vi "UHR-Fleezers Control (host) - 10.7.vi"() -> ()   [LabVIEW 2011] (continued)
            n774 = property on="Trap Delta (MHz)" class="DigNum (strict)"("Val(Sgnl)"="Trap Delta Before Moving") -> ()  [unwired: 2 in, 2 out]
          }
          frame #1 {
            n775 = local read "Saved Stage Positions"() -> (w1216:dbl[][])
            n776 = local write "FB Trap Pos Offset"(0.0 ("FB Trap Pos Offset")) -> ()
            n777 = property on="Trap Pos. FB Offset Factor" class="DigNum (strict)"("Val(Sgnl)"=i64 0 ("Value (Signaling)")) -> ()  [unwired: 2 in, 2 out]
            n778 = local write "Stage Moving"(TRUE ("Stage Moving")) -> ()
            n779 = call "move to saved stage position.vi"("error in"=w1213, "Stage VISA resource name in"=w1214, "Position"="Stage Position To Establish FB", "Saved Stage Positions"=w1216) -> ("error out"=w1212:errorcluster)  [unwired: 1 out]
            n780 = local write "Stage Control Serial Error"(w1212) -> ()
          }
          frame #2 {
            n781 = call <vilib>:"Beep.vi"() -> ()  [unwired: 3 in, 9 out]
            n782 = Multiply(x="Wait (s)", y=u32 1000 ("milliseconds to wait")) -> (x*y=w1222:u32)
            n783 = property on="Trap Delta (MHz)" class="DigNum (strict)"("Val(Sgnl)"="Starting \nTrap Delta (MHz)") -> ()  [unwired: 2 in, 2 out]
            n784 = local write "Stage Moving"(FALSE ("Stage Moving")) -> ()
            n785 = Wait (ms)(milliseconds to wait=w1222) -> ()  [unwired: 1 out]
            n786 = property on="Tab Control 2" class="TabCtl (strict)"("Val(Sgnl)"=T6."Feedback on Trap Position" ("Value (Signaling)")) -> ()  [unwired: 2 in, 2 out]
            n787 = property on="Tab Control" class="TabCtl (strict)"("Val(Sgnl)"=T4."Trap Control (RF)" ("Value (Signaling)")) -> ()  [unwired: 2 in, 2 out]
          }
          frame #3 {
            n788 = property on="Set Reading to\nSetpoint" class="Bool (strict)"("Val(Sgnl)"=TRUE ("Value (Signaling)")) -> ()  [unwired: 2 in, 2 out]
            n789 = Wait (ms)(milliseconds to wait=u32 500) -> ()  [unwired: 1 out]
          }
          frame #4 {
            n790 = property on="Trap Pos. FB ON" class="Bool (strict)"("Val(Sgnl)"=TRUE ("Value (Signaling)")) -> ()  [unwired: 2 in, 2 out]
            n791 = Wait (ms)(milliseconds to wait=u32 250) -> ()  [unwired: 1 out]
          }
          frame #5 {
            n792 = case shown="False" "Trap Trig Fl." {
              frame False {
                n793 = case shown="True" "Green ON after FB ON?" {
                  selector: "Green ON after FB ON?" -> [_ w1238]
                  frame False {
                  }
                  frame True {
                    n794 = property on="Green Laser ON/Interlacing" class="Bool (strict)"("Val(Sgnl)"=w1238) -> ()  [unwired: 2 in, 2 out]
                  }
                }
              }
              frame True {
              }
            }
            n795 = case shown="True" "Remove Action Offset" {
              tunnel: TRUE ("Value (Signaling)") -> [w1235 w1236]
              frame False {
                n796 = property on="Remove Unwinding Offset" class="Bool (strict)"("Val(Sgnl)"=w1235) -> ()  [unwired: 2 in, 2 out]
              }
              frame True {
                n797 = property on="Remove Action Offset" class="Bool (strict)"("Val(Sgnl)"=w1236) -> ()  [unwired: 2 in, 2 out]
              }
            }
            n798 = Wait (ms)(milliseconds to wait=u32 250) -> ()  [unwired: 1 out]
          }
          frame #6 {
            n799 = property on="Start Saving" class="Bool (strict)"("Val(Sgnl)"=TRUE ("Value (Signaling)")) -> ()  [unwired: 2 in, 2 out]
            n800 = Wait (ms)(milliseconds to wait=u32 5000) -> ()  [unwired: 1 out]
          }
          frame #7 {
            w1242 = TRUE ("Value (Signaling)")
            n801 = property on="Rem fb disp offset" class="Bool (strict)"("Val(Sgnl)"=w1242) -> ()  [unwired: 2 in, 2 out]
            n802 = property on="Remove Offset" class="Bool (strict)"("Val(Sgnl)"=w1242) -> ()  [unwired: 2 in, 2 out]
            n803 = Wait (ms)(milliseconds to wait=u32 100) -> ()  [unwired: 1 out]
          }
          frame #8 {
            n804 = case shown="True" w1245 {
              frame False {
              }
              frame True {
                n805 = local write "Trap Trig. Fl."(TRUE ("Value (Signaling)")) -> ()
              }
            }
          }
          frame #9 {
            n806 = case shown="True" "Start dipping after?" {
              frame False {
              }
              frame True {
                n807 = flat-sequence {
                  frame #0 {
                    n808 = Multiply(x="Delay before dipping (s)", y=1000.0) -> (x*y=w1249:dbl)
                    n809 = Wait (ms)(milliseconds to wait=w1249) -> ()  [unwired: 1 out]
                  }
                  frame #1 {
                    n810 = property on="Dip for Protein" class="Bool (strict)"("Val(Sgnl)"=TRUE ("Value (Signaling)")) -> ()  [unwired: 2 in, 2 out]
                    n811 = local write "Scripts"(T1."Dipping" ("Scripts")) -> ()
                  }
                }
              }
            }
          }
        }
      }
      event "Fixed Traps Data\nScript": Value Change {
        n812 = event-data() -> ()  [unwired: 1 in, 5 out]
        n813 = flat-sequence {
          frame #0 {
            n814 = case shown="True" "Green ON" {
              frame False {
              }
              frame True {
                n815 = property on="Green Laser ON/Interlacing" class="Bool (strict)"("Val(Sgnl)"=TRUE) -> ()  [unwired: 2 in, 2 out]
              }
            }
            n816 = local write "Offset (nm)"(0.0 ("Offset (nm)")) -> ()
            n817 = property on="Sample Channel\nFlow" class="Bool (strict)"("Val(Sgnl)"=FALSE ("Value (Signaling)")) -> ()  [unwired: 2 in, 2 out]
            n818 = property on="Trap Delta (MHz)" class="DigNum (strict)"("Val(Sgnl)"="Fixed Traps Trap Delta (MHz)") -> ()  [unwired: 2 in, 2 out]
          }
          frame #1 {
            n819 = Wait (ms)(milliseconds to wait=u32 1000) -> ()  [unwired: 1 out]
          }
          frame #2 {
            n820 = local write "Start Saving"(TRUE ("Start Saving")) -> ()
          }
          frame #3 {
            n821 = local read "Bead Sep. Int. Time (s)"() -> (w1260:dbl)
            n822 = Multiply(x=w1260, y=1000.0) -> (x*y=w1262:dbl)
            n823 = Wait (ms)(milliseconds to wait=w1262) -> ()  [unwired: 1 out]
          }
          frame #4 {
            n824 = property on="Remove Offset" class="Bool (strict)"("Val(Sgnl)"=TRUE ("Value (Signaling)")) -> ()  [unwired: 2 in, 2 out]
          }
          frame #5 {
            n825 = property on="Dip for Protein" class="Bool (strict)"("Val(Sgnl)"="Start dipping after?") -> ()  [unwired: 2 in, 2 out]
          }
        }
      }
      event "Got DNA bead": Value Change {
        n826 = event-data() -> ()  [unwired: 1 in, 5 out]
        n827 = flat-sequence {
          frame #0 {
            n828 = local read "Daq spot flow on"() -> (w1267:bool)
            n829 = case shown="True" w1267 {
              frame False {
              }
              frame True {
                n830 = property on="Sample Channel\nFlow" class="Bool (strict)"("Val(Sgnl)"=TRUE ("Value (Signaling)")) -> ()  [unwired: 2 in, 2 out]
              }
            }
            n831 = property on="Got DNA bead" class="Bool"("Key Focus"=FALSE) -> ()  [unwired: 2 in, 2 out]
          }
          frame #1 {
            n832 = property on="Inject Pump 1" class="Bool (strict)"("Val(Sgnl)"=FALSE ("Value (Signaling)")) -> ()  [unwired: 2 in, 2 out]
          }
          frame #2 {
            n833 = property on="Cal/Data Acq. Spot" class="Bool (strict)"("Val(Sgnl)"=TRUE ("Value (Signaling)")) -> ()  [unwired: 2 in, 2 out]
          }
        }
      }
      event "Take Stepping Data": Value Change {
        n834 = event-data() -> ()  [unwired: 1 in, 5 out]
        n835 = local read "Save ave N"() -> (w1279:dbl)
        n836 = flat-sequence {
          tunnel: w1279 -> [w1281]
          tunnel: [w1281] -> w1274
          tunnel: [w1283] -> w1275
          tunnel: w1274 -> [w1283]
          tunnel: [w1285] -> w1276
          tunnel: w1275 -> [w1285]
          tunnel: [w1288] -> w1277
          tunnel: w1276 -> [w1288]
          tunnel: [w1290] -> w1278
          tunnel: w1277 -> [w1290]
          tunnel: [w1292] -> w1272
          tunnel: w1278 -> [w1292]
          tunnel: w1272 -> [w1295]
          tunnel: [w1295] -> w1271
          tunnel: w1271 -> [w1296]
          tunnel: [w1296] -> w1273
          tunnel: w1273 -> [w1302]
          frame #0 {
            n837 = property on="Save ave N" class="DigNum (strict)"("Val(Sgnl)"="Save ave factor") -> ()  [unwired: 2 in, 2 out]
          }
          frame #1 {
            n838 = Wait (ms)(milliseconds to wait=u32 100) -> ()  [unwired: 1 out]
          }
          frame #2 {
            n839 = local read "Offset 2 Start (MHz)"() -> (w1287:dbl)
            n840 = property on="Saved AOD Raster Scan Parameter Sets" class="Arr (strict)"("Index Values"=u32[] [2]) -> ()  [unwired: 2 in, 2 out]
            n841 = property on="Trap Delta (MHz)" class="DigNum (strict)"("Val(Sgnl)"=w1287) -> ()  [unwired: 2 in, 2 out]
          }
          frame #3 {
            n842 = property on="Load parameters" class="Bool (strict)"("Val(Sgnl)"=TRUE ("Value (Signaling)")) -> ()  [unwired: 2 in, 2 out]
          }
          frame #4 {
            n843 = Wait (ms)(milliseconds to wait=u32 100) -> ()  [unwired: 1 out]
          }
          frame #5 {
            n844 = property on="Trap Raster Scan" class="Bool (strict)"("Val(Sgnl)"=TRUE ("Value (Signaling)")) -> ()  [unwired: 2 in, 2 out]
          }
          frame #6 {
            n845 = Wait (ms)(milliseconds to wait=u32 1000) -> ()  [unwired: 1 out]
          }
          frame #7 {
            n846 = while {
              stop <- w1299 stop-if-true
              n847 = local read "Raster Scanning..."() -> (w1301:bool)
              n848 = local read "Saving..."() -> (w1300:bool)
              n849 = Not(x=w1300) -> (.not. x?=w1297:bool)
              n850 = Not(x=w1301) -> (.not. x?=w1298:bool)
              n851 = And(x=w1298, y=w1297) -> (x .and. y?=w1299:bool)
            }
          }
          frame #8 {
            n852 = property on="Save ave N" class="DigNum (strict)"("Val(Sgnl)"=w1302) -> ()  [unwired: 2 in, 2 out]
          }
        }
      }
      event "Step Size (nm)": Value Change {
        n853 = event-data() -> ()  [unwired: 1 in, 5 out]
        n854 = flat-sequence {
          frame #0 {
            n855 = property on="Saved AOD Raster Scan Parameter Sets" class="Arr (strict)"("Index Values"=u32[] [1]) -> ()  [unwired: 2 in, 2 out]
          }
          frame #1 {
            n856 = Multiply(x="N Steps", y="Step Size (nm)") -> (x*y=w1304:dbl)
            n857 = property on="Scan Speed AOD (nm/s) 2" class="DigNum (strict)"("Value"="Step Size (nm)") -> ()  [unwired: 2 in, 2 out]
            n858 = property on="Step Size AOD (nm) 2" class="DigNum (strict)"("Value"="Step Size (nm)") -> ()  [unwired: 2 in, 2 out]
            n859 = property on="Scan Range AOD (nm) 2" class="DigNum (strict)"("Value"=w1304) -> ()  [unwired: 2 in, 2 out]
          }
        }
      }
      event "Take Detection Laser\nImage": Value Change {
        n860 = event-data() -> ()  [unwired: 1 in, 5 out]
        n861 = flat-sequence {
          tunnel: [w1332] -> w1322
          tunnel: [w1331] -> w1315
          tunnel: [w1330] -> w1307
          tunnel: [w1335] -> w1323
          tunnel: w1322 -> [w1335]
          tunnel: [w1334] -> w1316
          tunnel: w1315 -> [w1334]
          tunnel: [w1333] -> w1308
          tunnel: w1307 -> [w1333]
          tunnel: [w1339] -> w1324
          tunnel: w1323 -> [w1339]
          tunnel: [w1338] -> w1317
          tunnel: w1316 -> [w1338]
          tunnel: [w1337] -> w1309
          tunnel: w1308 -> [w1337]
          tunnel: [w1345] -> w1325
          tunnel: w1324 -> [w1345]
          tunnel: [w1344] -> w1318
          tunnel: w1317 -> [w1344]
          tunnel: [w1343] -> w1310
          tunnel: w1309 -> [w1343]
          tunnel: [w1349] -> w1326
          tunnel: w1325 -> [w1349]
          tunnel: [w1348] -> w1319
          tunnel: w1318 -> [w1348]
          tunnel: [w1347] -> w1311
          tunnel: w1310 -> [w1347]
          tunnel: [w1353] -> w1327
          tunnel: w1326 -> [w1353]
          tunnel: [w1352] -> w1320
          tunnel: w1319 -> [w1352]
          tunnel: [w1351] -> w1312
          tunnel: w1311 -> [w1351]
          tunnel: [w1357] -> w1328
          tunnel: w1327 -> [w1357]
          tunnel: [w1356] -> w1321
          tunnel: w1320 -> [w1356]
          tunnel: [w1355] -> w1313
          tunnel: w1312 -> [w1355]
          tunnel: w1328 -> [w1363]
          tunnel: w1321 -> [w1362]
          tunnel: [w1360] -> w1314
          tunnel: w1313 -> [w1360]
          tunnel: w1314 -> [w1364]
          frame #0 {
            n862 = local read "Green Laser ON/Interlacing"() -> (w1332:bool)
            n863 = local read "Green laser mode"() -> (w1331:enum32{"Laser ON", "Laser OFF", "Interlace"})
            n864 = local read "Green FB On/Off"() -> (w1330:bool)
          }
          frame #1 {
            n865 = property on="Green FB On/Off" class="Bool (strict)"("Val(Sgnl)"=FALSE ("Value (Signaling)")) -> ()  [unwired: 2 in, 2 out]
          }
          frame #2 {
            n866 = property on="Green Laser ON/Interlacing" class="Bool (strict)"("Val(Sgnl)"=TRUE ("Value (Signaling)")) -> ()  [unwired: 2 in, 2 out]
            n867 = property on="Flip Green Filter" class="Bool (strict)"("Val(Sgnl)"=TRUE ("Value (Signaling)")) -> ()  [unwired: 2 in, 2 out]
            n868 = property on="Green laser mode" class="RadioBtnsControl (strict)"("Val(Sgnl)"=enum32{"Laser ON", "Laser OFF", "Interlace"}."Laser ON" ("Value (Signaling)")) -> ()  [unwired: 2 in, 2 out]
          }
          frame #3 {
            n869 = Wait (ms)(milliseconds to wait=u32 500) -> ()  [unwired: 1 out]
          }
          frame #4 {
            n870 = property on="Confocal Image" class="Bool (strict)"("Val(Sgnl)"=TRUE ("Value (Signaling)")) -> ()  [unwired: 2 in, 2 out]
          }
          frame #5 {
            n871 = Wait (ms)(milliseconds to wait=u32 2000) -> ()  [unwired: 1 out]
          }
          frame #6 {
            n872 = while {
              stop <- w1358 stop-if-true
              n873 = local read "Saving..."() -> (w1359:bool)
              n874 = Not(x=w1359) -> (.not. x?=w1358:bool)
            }
          }
          frame #7 {
            n875 = property on="Flip Green Filter" class="Bool (strict)"("Val(Sgnl)"=TRUE ("Value (Signaling)")) -> ()  [unwired: 2 in, 2 out]
            n876 = property on="Green Laser ON/Interlacing" class="Bool (strict)"("Val(Sgnl)"=w1363) -> ()  [unwired: 2 in, 2 out]
            n877 = property on="Green laser mode" class="RadioBtnsControl (strict)"("Val(Sgnl)"=w1362) -> ()  [unwired: 2 in, 2 out]
          }
          frame #8 {
            n878 = property on="Green FB On/Off" class="Bool (strict)"("Val(Sgnl)"=w1364) -> ()  [unwired: 2 in, 2 out]
          }
        }
      }
      event "Stop All": Value Change {
        n879 = event-data() -> ()  [unwired: 1 in, 5 out]
        n880 = local read "Stop All"() -> (w1365:bool)
      }
    }
    n881 = node-c288() -> ()  [unwired: 1 in, 1 out]
  }
  n882 = node-c288(2 ("Processor")) -> (w92:T21)  [unwired: 3 out]
  n883 = node-c288() -> (w94:T21)  [unwired: 4 out]
  n884 = timed-loop "Control parameters (event loop)" {
    tunnel: w50 -> [w1374]
    shift-right: [w1373] -> _
    shift-left: errorcluster {"status"=FALSE, "code"=0, "source"=""} ("error out") -> [w1372]
    tunnel: [w1371] -> _
    timing: w92 -> [_]
    timing-out: [_] -> w91
    tunnel: w64 -> [w1370]
    tunnel: w4 -> [w1369]
    tunnel: w3 -> [w1368]
    tunnel: w2 -> [w1367]
    tunnel: w1 -> [w1366]
    stop <- w1371 stop-if-true
    n885 = node-c288() -> ()  [unwired: 2 out]
    n886 = event shown="[56] \"Retract Pump 3\": Value Change" {
      selector: _ -> [_ _ _ _ _ _ _ _ _ _ _ _ _ _ _ _ _ _ _ _ _ _ _ _ _ _ _ _ _ _ _ _ _ _ _ _ _ _ _ _ _ _ _ _ _ _ _ _ _ _ _ _ _ _ _ _ _ _ _ _ _ _ _ _ _ _ _ _ _ _ _ _ _]
      dyn-events: _ -> [_ _ _ _ _ _ _ _ _ _ _ _ _ _ _ _ _ _ _ _ _ _ _ _ _ _ _ _ _ _ _ _ _ _ _ _ _ _ _ _ _ _ _ _ _ _ _ _ _ _ _ _ _ _ _ _ _ _ _ _ _ _ _ _ _ _ _ _ _ _ _ _ _]
      timeout: _ -> [_ _ _ _ _ _ _ _ _ _ _ _ _ _ _ _ _ _ _ _ _ _ _ _ _ _ _ _ _ _ _ _ _ _ _ _ _ _ _ _ _ _ _ _ _ _ _ _ _ _ _ _ _ _ _ _ _ _ _ _ _ _ _ _ _ _ _ _ _ _ _ _ _]
      tunnel: w1374 -> [w1412 _ _ _ w1450 _ w1472 _ _ _ _ w1538 _ _ w1581 w1587 w1592 w1598 w1634 w1652 w1659 w1670 w1674 w1685 w1696 w1707 w1718 w1729 w1740 w1767 w1861 w1868 w1906 _ w1941 w1945 w1956 w1960 w1964 _ w1972 _ _ _ _ _ _ _ _ _ _ _ _ _ _ _ _ _ w2350 _ w2367 _ w2374 w2392 _ w2399 w2407 w2422 w2433 w2436 w2441 _ w2460]
      tunnel: [w1411 _ _ _ w1440 _ w1471 _ _ w1503 _ w1517 _ _ w1580 w1583 w1589 w1595 w1633 w1650 w1658 w1668 _ w1679 w1690 w1701 w1712 w1723 w1734 w1765 w1859 w1866 w1904 _ w1939 w1943 w1946 w1958 w1962 _ w1970 _ _ _ _ _ _ _ _ _ _ _ _ _ _ _ _ _ w2348 _ _ _ _ w2389 _ _ _ _ _ _ _ _ _] -> w1373
      tunnel: w1372 -> [w1410 _ _ _ w1449 _ w1470 _ _ w1503 _ w1537 _ _ w1579 w1582 w1588 w1594 w1632 w1651 w1657 w1669 w1673 w1684 w1695 w1706 w1717 w1728 w1739 w1766 w1860 w1867 w1905 _ w1940 w1944 w1955 w1959 w1963 _ w1971 _ _ _ _ _ _ _ _ _ _ _ _ _ _ _ _ _ w2349 _ w2366 _ w2373 w2391 _ w2398 w2406 w2421 w2432 w2435 w2440 _ w2459]
      tunnel: [_ _ _ _ _ _ _ _ _ w1502 _ _ _ _ _ _ _ _ _ _ _ _ _ _ _ _ _ _ _ _ _ _ _ _ _ _ _ _ _ _ _ _ _ _ _ _ _ _ _ _ _ _ _ _ _ _ _ _ _ _ _ _ _ _ _ _ _ _ _ _ _ _ _] -> w1371
      tunnel: [_ _ _ _ _ _ _ "Round T1 X" _ _ _ _ _ _ _ _ _ _ _ _ _ _ _ _ _ _ _ _ _ _ _ _ _ _ _ _ _ _ _ _ _ _ _ _ _ _ _ _ _ _ _ _ _ _ _ _ _ _ _ _ _ _ _ _ _ _ _ _ _ _ _ _ _] -> _
      tunnel: [_ _ _ "Adjust Scale\nto Mean" _ _ _ _ _ _ _ _ _ _ _ _ _ _ _ _ _ "Test ttrig" _ _ _ _ _ _ _ _ _ _ _ _ _ _ _ _ _ _ _ _ _ _ _ _ _ _ "Flush Sample" "Flush Pump 3" "Flush Pump 1" "Clear Volume" _ _ _ _ _ _ _ _ _ _ _ _ _ _ _ _ _ _ _ _ _] -> _
      tunnel: [_ _ _ _ _ _ _ _ "Round T2 X" _ "Delayed Interlace Start" _ _ _ _ _ _ _ _ _ _ _ _ _ _ _ _ _ _ _ _ _ _ _ _ _ _ _ _ _ _ _ _ _ _ _ _ _ _ _ _ _ _ _ _ _ _ _ _ _ _ _ _ _ _ _ _ _ _ _ _ _ _] -> _
      tunnel: w1370 -> [_ _ _ _ _ _ _ _ _ _ _ _ _ _ _ _ _ _ _ _ _ _ _ _ _ _ _ _ _ _ _ _ _ _ _ _ _ _ _ _ _ _ _ _ w2129 w2136 w2143 w2148 w2157 _ _ w2263 _ _ _ _ _ _ _ _ _ _ _ _ _ _ _ _ _ _ _ _ _]
      tunnel: w1369 -> [_ _ _ _ _ _ _ _ _ _ _ _ _ _ _ _ _ _ _ _ _ _ _ _ _ _ _ _ _ _ _ _ _ _ _ _ _ _ _ _ _ _ w2046 _ _ _ _ _ _ w2201 _ _ w2269 _ w2278 _ w2292 _ _ _ _ _ _ _ _ _ _ _ _ _ _ _ _]
      tunnel: w1368 -> [_ _ _ _ _ _ _ _ _ _ _ _ _ _ _ _ _ _ _ _ _ _ _ _ _ _ _ _ _ _ _ _ _ _ _ _ _ _ _ _ _ _ _ _ _ _ _ _ _ _ _ _ _ _ _ _ _ _ _ _ _ _ _ _ _ _ _ _ _ _ _ _ _]
      tunnel: w1367 -> [_ _ _ _ _ _ _ _ _ _ _ _ _ _ _ _ _ _ _ _ _ _ _ _ _ _ _ _ _ _ _ _ _ _ _ _ _ _ _ _ _ w1983 _ _ _ _ _ _ _ _ w2231 _ _ w2274 _ w2285 _ w2317 _ _ _ _ _ _ _ _ _ _ _ _ _ _ _]
      tunnel: w1366 -> [_ _ _ _ _ _ _ _ _ _ _ _ _ _ _ _ _ _ _ _ _ _ _ _ _ _ _ _ _ _ _ _ _ _ _ _ _ _ _ _ _ _ _ _ _ _ _ _ _ _ _ _ _ _ _ _ _ _ _ _ _ _ _ _ _ _ _ _ _ _ _ _ _]
      event "AI Count (ticks)", "Sets to FIFO (Traps)", "Save ave N", "FPGA Ave.", "# Samples/channel", "N sets to save": Value Change {
        # "So that if 'Save ave N' is updated, the AOD scanning code updates too."
        n887 = event-data() -> ()  [unwired: 6 out]
        n888 = local read "AI Count (ticks)"() -> (w1392:u32)
        n889 = Boolean To (0,1)(Boolean="Sets to FIFO (Traps)") -> (0, 1=w1402:cluster{"Set 1":i16, "Set 2":i16, "Set 3":i16})
        n890 = xnode "Read/Write Control"("FPGA VI Reference In"=w1412, "error in"=w1410, "ai count"=w1392, "AI1 Sets to FIFO"="Sets to FIFO (Traps)", "N of AI1 Int Acq Sets"="N Acq Sets (Traps + Fl.)") -> ("error out"=w1411:errorcluster)  [unwired: 1 out]
        n891 = Cluster To Array(cluster=w1402) -> (array=w1401:i16[])
        n892 = To Unsigned Long Integer(number=w1401) -> (unsigned 32bit integer=w1381:u32[])
        n893 = local read "Scan steps (AOD)"() -> (w1403:u64)
        n894 = Multiply(x=w1392, y="N Acq Sets (Traps + Fl.)") -> (x*y=w1390:u32)
        n895 = Divide(x=40000000.0, y=w1392) -> (x/y=w1384:dbl)
        "AI rate (Hz)" <- w1384
        "Ave. Rate (Hz)" <- w1384
        n896 = Add Array Elements(numeric array=w1381) -> (sum=w1393:u32)
        "Trap Sets" <- w1393
        n897 = Reciprocal(x=w1384) -> (1/x=→"Ave. Period (s)":dbl)
        n898 = property on="Scan steps (AOD)" class="DigNum (strict)"("Val(Sgnl)"=w1403) -> ()  [unwired: 2 in, 2 out]
        n899 = Divide(x=w1384, y="N Acq Sets (Traps + Fl.)") -> (x/y=w1407:dbl)
        "Data Rate (Hz)" <- w1407
        n900 = Reciprocal(x=w1407) -> (1/x=→"Data Period (s)":dbl)
        n901 = local read "Save ave N"() -> (w1406:dbl)
        n902 = Divide(x=w1407, y=w1406) -> (x/y=w1405:dbl)
        "Save Data Rate (Hz)" <- w1405
        n903 = Reciprocal(x=w1405) -> (1/x=→"Save Data Period (s)":dbl)
        n904 = Multiply(x=w1390, y="# Samples/trap") -> (x*y=w1388:u32)
        "Counts/DMA" <- w1388
        n905 = property on="Trap Disp. Downsample" class="DigNum (strict)"("Maximum"="# Samples/trap") -> ()  [unwired: 2 in, 2 out]
        n906 = Multiply(x=w1393, y="# Samples/trap") -> (x*y=w1382:u32)
        "# Samples/channel" <- w1382
        n907 = Multiply(x=w1382, y=u32 8) -> (x*y=→"Trap AI Elements/DMA read":u32)
        n908 = local read "APD Int. Count"() -> (w1389:u32)
        n909 = Multiply(x=w1382, y=u32 3) -> (x*y=→"Trap Pos Elements/DMA read":u32)
        n910 = Divide(x=w1388, y=w1389) -> (x/y=w1379:dbl)
        "APD Samples/FIFO Acq." <- w1379
        n911 = Divide(x=w1388, y=40000000.0) -> (x/y=w1386:dbl)
        "DMA Update Period (s)" <- w1386
        n912 = Multiply(x=2.0, y=w1379) -> (x*y=→"APD Elements/DMA read":dbl)
        n913 = property on="APD Disp. Downsample" class="DigNum (strict)"("Maximum"=w1379) -> ()  [unwired: 2 in, 2 out]
        n914 = local read "N sets to save"() -> (w1399:u32)
        n915 = Multiply(x=w1386, y=w1399) -> (x*y=→"Total Time (s)":dbl)
        "FPGA Averaging" <- FALSE ("FPGA Averaging")
      }
      event "Remove Offset": Value Change {
        n916 = event-data() -> ()  [unwired: 7 out]
        n917 = local write "Remove Offset"(FALSE ("Remove Offset")) -> ()
        n918 = local read "Bead Mean (nm)"() -> (w1414:dbl)
        n919 = local read "Offset (nm)"() -> (w1415:dbl)
        n920 = Add(x=w1414, y=w1415) -> (x+y=w1413:dbl)
        n921 = local write "Offset (nm)"(w1413) -> ()
        n922 = disable-structure shown="Disabled" {
          frame Disabled {
            n923 = local read "Bead Mean (nm)"() -> (w1420:dbl)
            n924 = Add(y=w1420) -> (x=w1419:dbl, x+y=w1418:dbl)
            n925 = Subtract(x=w1420, y=w1419) -> (x-y=w1417:dbl)
            n926 = property on="Bead Separation" class="WFChart (strict)"("YScale.Minimum"=w1417) -> ()  [unwired: 2 in, 2 out]
            n927 = property on="Bead Separation" class="WFChart (strict)"("YScale.Maximum"=w1418) -> ()  [unwired: 2 in, 2 out]
          }
          frame Enabled {
          }
        }
      }
      event "Detector Type": Value Change {
        n928 = event-data() -> ()  [unwired: 7 out]
        n929 = local read "AI labels"() -> (w1421:string[])
        n930 = property on="High Res. Display" class="Ring (strict)"("Strings []"=w1421) -> ()  [unwired: 2 in, 2 out]
        n931 = Build Array (concatenate)(w1421, "none") -> (w1422:string[])
        n932 = property on="FFT 1 Choice 1" class="Ring (strict)"("Strings []"=w1422) -> ()  [unwired: 2 in, 2 out]
        n933 = property on="FFT 1 Choice 2" class="Ring (strict)"("Strings []"=w1422) -> ()  [unwired: 2 in, 2 out]
        n934 = property on="FFT 2 Choice 1" class="Ring (strict)"("Strings []"=w1422) -> ()  [unwired: 2 in, 2 out]
        n935 = property on="FFT 2 Choice 2" class="Ring (strict)"("Strings []"=w1422) -> ()  [unwired: 2 in, 2 out]
        n936 = Bundle("APD 1", "APD 2") -> (w1425:cluster{string, string})  [unwired: 1 out]
        n937 = Cluster To Array(cluster=w1425) -> (array=w1423:string[])
        n938 = Build Array (concatenate)(w1423, w1422) -> (w1427:string[])
        n939 = Array Size(array=w1427) -> (size(s)=w1428:i32)
        n940 = property on="Signals to Plot" class="LstBox (strict)"("Item Names"=w1427) -> ()  [unwired: 2 in, 2 out]
        n941 = property on="Signals to Plot" class="LstBox (strict)"("Number of Rows"=w1428) -> ()  [unwired: 2 in, 2 out]
        n942 = property on="All Signals" class="WFChart (strict)"("LegNumRows"=w1428) -> ()  [unwired: 2 in, 2 out]
      }
      event "Adjust Scale\nto Mean": Value Change {
        n943 = event-data() -> ()  [unwired: 7 out]
        n944 = local read "APD 1 Rate (Hz)"() -> (w1437:dbl)
        n945 = Multiply(x=1000.0, y="Above (kHz)") -> (x*y=w1435:dbl)
        n946 = Multiply(x=1000.0, y="Below (kHz)") -> (x*y=w1433:dbl)
        n947 = Add(x=w1435, y=w1437) -> (x+y=w1430:dbl)
        n948 = Subtract(x=w1437, y=w1433) -> (x-y=w1431:dbl)
        n949 = property on="APD Chart" class="WFChart (strict)"("YScale.Minimum"=w1431) -> ()  [unwired: 2 in, 2 out]
        n950 = property on="APD Chart" class="WFChart (strict)"("YScale.Maximum"=w1430) -> ()  [unwired: 2 in, 2 out]
      }
      event "Phase adj. (AI1)", "+ phase (AI1)", "- phase (AI1)": Value Change {
        n951 = event-data() -> ()  [unwired: 7 out]
        n952 = Negate(x="Phase adj. (AI1)") -> (-x=w1447:i16)
        n953 = Select(t=w1447, s="- phase (AI1)", f="Phase adj. (AI1)") -> (s? t:f=w1446:i16)
        n954 = xnode "Read/Write Control"("FPGA VI Reference In"=w1450, "error in"=w1449, "Phase count adjustment"=w1446) -> ("FPGA VI Reference Out"=w1445:T19, "error out"=w1444:errorcluster)
        n955 = Or(x="- phase (AI1)", y="+ phase (AI1)") -> (x .or. y?=w1441:bool)
        n956 = xnode "Read/Write Control"("FPGA VI Reference In"=w1445, "error in"=w1444, "+ phase"=w1441) -> ("error out"=w1440:errorcluster)  [unwired: 1 out]
      }
      event "Signals to Plot": Double Click {
        w1453 = u32 9868950 ("Color Box")
        n957 = event-data() -> ("Row"=w1455:i32)  [unwired: 9 out]
        n958 = property on="All Signals" class="WFChart (strict)"("Active Plot"=w1455) -> (error out=w1466:errorcluster)  [unwired: 2 in, 1 out]
        n959 = property on="All Signals" class="WFChart (strict)" props=["Plot", "Visible?", "Plot", "Plot Color"](error in=w1466) -> (error out=w1465:errorcluster, "Plot.Visible?"=w1464:bool)  [unwired: 1 in, 2 out]
        n960 = Select(t=FALSE ("Plot.Visible"), s=w1464, f=TRUE ("Plot.Visible")) -> (s? t:f=w1459:bool)
        n961 = property on="All Signals" class="WFChart (strict)"(error in=w1465, "Plot.Visible?"=w1459) -> (error out=w1461:errorcluster)  [unwired: 1 in, 1 out]
        n962 = property on="All Signals" class="WFChart (strict)"(error in=w1461) -> (error out=w1456:errorcluster, "Plot.Plot Color"=w1460:u32)  [unwired: 1 in, 1 out]
        n963 = property on="Signals to Plot" class="LstBox (strict)"(error in=w1456, "Active Row"=w1455) -> (error out=w1454:errorcluster)  [unwired: 1 in, 1 out]
        n964 = Select(t=w1460, s=w1459, f=u32 0) -> (s? t:f=w1457:u32)
        n965 = property on="Signals to Plot" class="LstBox (strict)"(error in=w1454, "CellFontColor"=w1457, "SelColor"=w1453, "CellBG"=w1453, "CellFontSize"=u32 20 ("Active Row:Cell Font:Size"), "CellFontBold"=TRUE ("Active Row:Cell Font:Bold")) -> ()  [unwired: 1 in, 2 out]
      }
      event "BD 1 Frequency 1 (MHz)", "BD 1 Frequency 2 (MHz)", "BD 1 Frequency 3 (MHz)", "BD 2 Frequency 1 (MHz)", "BD 2 Frequency 2 (MHz)", "BD 2 Frequency 3 (MHz)", "Trap Delta (MHz)": Value Change {
        n966 = event-data() -> ("CtlRef"=w1469:refnum<vi>)  [unwired: 6 out]
        n967 = control-ref of="Trap Delta (MHz)"() -> (w1468:refnum<vi>)
        n968 = Equal?(x=w1468, y=w1469) -> (x = y?=w1467:bool)
        n969 = case shown="False" "Oscillate Set 1" {
          tunnel: w1472 -> [w1492 _]
          tunnel: [w1491 w1495] -> w1471
          tunnel: w1470 -> [w1490 w1495]
          tunnel: w1467 -> [w1475 _]
          frame False {
            n970 = local read "BD 1 Frequency 2 (MHz)"() -> (w1479:dbl)
            n971 = local read "BD 1 Frequency 1 (MHz)"() -> (w1477:dbl)
            n972 = Subtract(x=w1479, y="Trap Delta (MHz)") -> (x-y=w1476:dbl)
            n973 = Select(t=w1476, s=w1475, f=w1477) -> (s? t:f=w1474:dbl)
            n974 = local read "Y RF Frequency Limits (MHz)"() -> (w1480:T16)
            n975 = local read "X RF Frequency Limits (MHz)"() -> (w1481:T16)
            n976 = local read "BD 1 Frequency 3 (MHz)"() -> (w1493:dbl)
            n977 = local write "BD 1 Frequency 1 (MHz)"(w1474) -> ()
            n978 = local read "BD 2 Frequency 1 (MHz)"() -> (w1484:dbl)
            n979 = local read "BD 2 Frequency 2 (MHz)"() -> (w1483:dbl)
            n980 = local read "BD 2 Frequency 3 (MHz)"() -> (w1494:dbl)
            n981 = call "set RF board frequency - interlace.vi"("Board 2 Frequency Limits"=w1480, "Board 1 Frequency Limits"=w1481, "error in"=w1490, "FPGA VI Reference In"=w1492, "Board 2 Frequency 3 (MHz)"=w1494, "Board 1 Frequency 3 (MHz)"=w1493, "Board 2 Frequency 2 (MHz)"=w1483, "Board 2 Frequency 1 (MHz)"=w1484, "Board 1 Frequency 2 (MHz)"=w1479, "Board 1 Frequency 1  (MHz)"=w1474) -> ("error out"=w1491:errorcluster)  [unwired: 1 out]
            n982 = Subtract(x=w1484, y=w1483) -> (x-y=w1488:dbl)
            n983 = Subtract(x=w1474, y=w1479) -> (x-y=w1489:dbl)
            n984 = Square(x=w1488) -> (x^2=w1486:dbl)
            n985 = Square(x=w1489) -> (x^2=w1487:dbl)
            n986 = Add(x=w1487, y=w1486) -> (x+y=w1485:dbl)
            n987 = Square Root(x=w1485) -> (sqrt(x)=w1482:dbl)
            n988 = local write "Trap Delta (MHz)"(w1482) -> ()
            n989 = property on="Initial delta (MHz)" class="DigNum (strict)"("Val(Sgnl)"=w1482) -> ()  [unwired: 2 in, 2 out]
          }
          frame True {
          }
        }
      }
      event "Round T1 X": Value Change {
        n990 = event-data() -> ()  [unwired: 7 out]
        n991 = local read "BD 1 Frequency 1 (MHz)"() -> (w1498:dbl)
        n992 = Round To Nearest(number=w1498) -> (nearest integer value=w1497:dbl)
        n993 = property on="BD 1 Frequency 1 (MHz)" class="DigNum (strict)"("Val(Sgnl)"=w1497) -> ()  [unwired: 2 in, 2 out]
      }
      event "Round T2 X": Value Change {
        n994 = event-data() -> ()  [unwired: 7 out]
        n995 = local read "BD 1 Frequency 2 (MHz)"() -> (w1500:dbl)
        n996 = Round To Nearest(number=w1500) -> (nearest integer value=w1499:dbl)
        n997 = property on="BD 1 Frequency 2 (MHz)" class="DigNum (strict)"("Val(Sgnl)"=w1499) -> ()  [unwired: 2 in, 2 out]
      }
      event "Stop All": Value Change {
        n998 = event-data() -> ()  [unwired: 7 out]
        n999 = local read "Stop All"() -> (w1502:bool)
      }
      event "Delayed Interlace Start": Value Change {
        n1000 = event-data() -> ()  [unwired: 7 out]
        n1001 = flat-sequence {
          frame #0 {
            n1002 = Multiply(x="Delay to Interlace (s)", y=1000.0) -> (x*y=w1505:dbl)
            n1003 = Wait (ms)(milliseconds to wait=w1505) -> ()  [unwired: 1 out]
          }
          frame #1 {
            n1004 = property on="Green laser mode" class="RadioBtnsControl (strict)"("Val(Sgnl)"=enum32{"Laser ON", "Laser OFF", "Interlace"}."Interlace" ("Value (Signaling)")) -> ()  [unwired: 2 in, 2 out]
          }
        }
      }
      event "BD 1 Amplitude 1 (%)", "BD 1 Amplitude 2 (%)", "BD 1 Amplitude 3 (%)", "BD 2 Amplitude 1 (%)", "BD 2 Amplitude 2 (%)", "BD 2 Amplitude 3 (%)", "Trap 1 ON", "Trap 2 ON", "Trap 3 ON", "Feedback On/Off", "All FB On/Off": Value Change {
        w1529 = i16 1 ("f")
        n1005 = event-data() -> ()  [unwired: 7 out]
        n1006 = local write "Trap 1 (ON/OFF)"("Trap 1 ON") -> ()
        n1007 = local write "Trap 2 (ON/OFF)"("Trap 2 ON") -> ()
        n1008 = Boolean To (0,1)(Boolean="Trap 3 ON") -> (0, 1=w1530:i16)
        n1009 = Boolean To (0,1)(Boolean="Trap 1 ON") -> (0, 1=w1531:i16)
        n1010 = Boolean To (0,1)(Boolean="Trap 2 ON") -> (0, 1=w1532:i16)
        n1011 = Select(t=w1532, s="Trap ON/OFF X or Y Amp?", f=w1529) -> (s? t:f=w1527:i16)
        n1012 = Select(t=w1531, s="Trap ON/OFF X or Y Amp?", f=w1529) -> (s? t:f=w1528:i16)
        n1013 = Select(t=w1530, s="Trap ON/OFF X or Y Amp?", f=w1529) -> (s? t:f=w1526:i16)
        n1014 = Select(t=w1529, s="Trap ON/OFF X or Y Amp?", f=w1532) -> (s? t:f=w1524:i16)
        n1015 = Select(t=w1529, s="Trap ON/OFF X or Y Amp?", f=w1531) -> (s? t:f=w1525:i16)
        n1016 = Select(t=w1529, s="Trap ON/OFF X or Y Amp?", f=w1530) -> (s? t:f=w1523:i16)
        n1017 = And(x="All FB On/Off", y="Feedback On/Off") -> (x .and. y?=w1521:cluster{"Set 1":bool, "Set 2":bool})
        n1018 = local read "BD 1 Amplitude 1 (%)"() -> (w1541:dbl)
        n1019 = local read "BD 1 Amplitude 2 (%)"() -> (w1540:dbl)
        n1020 = local read "BD 1 Amplitude 3 (%)"() -> (w1539:dbl)
        n1021 = Unbundle By Name(w1521) -> ("Set 1"=w1516:bool, "Set 2"=w1513:bool)
        n1022 = local read "Y RF Amplitude Limits (%)"() -> (w1509:T16)
        n1023 = local read "X RF Amplitude Limits (%)"() -> (w1510:T16)
        n1024 = local read "BD 2 Amplitude 1 (%)"() -> (w1542:dbl)
        n1025 = local read "BD 2 Amplitude 2 (%)"() -> (w1543:dbl)
        n1026 = local read "BD 2 Amplitude 3 (%)"() -> (w1544:dbl)
        n1027 = And(x="Trap 2 ON", y=w1513) -> (x .and. y?=w1511:bool)
        n1028 = And(x="Trap 1 ON", y=w1516) -> (x .and. y?=w1514:bool)
        n1029 = Multiply(x=w1528, y=w1541) -> (x*y=w1536:dbl)
        n1030 = Multiply(x=w1540, y=w1527) -> (x*y=w1534:dbl)
        n1031 = Multiply(x=w1539, y=w1526) -> (x*y=w1535:dbl)
        n1032 = Multiply(x=w1542, y=w1525) -> (x*y=w1545:dbl)
        n1033 = Multiply(x=w1543, y=w1524) -> (x*y=w1546:dbl)
        n1034 = Multiply(x=w1544, y=w1523) -> (x*y=w1547:dbl)
        n1035 = call "set RF board amplitude - interlace.vi"("Board 2 Amplitude Limits"=w1509, "Board 1 Amplitude Limits"=w1510, "error in"=w1537, "FPGA VI Reference In"=w1538, "Board 2 Amplitude 3 (%)"=w1547, "Board 1 Amplitude 3 (%)"=w1535, "Board 2 Amplitude 2 (%)"=w1546, "Board 2 Amplitude 1 (%)"=w1545, "Board 1 Amplitude 2 (%)"=w1534, "Board 1 Amplitude 1 (%)"=w1536) -> ("error out"=w1518:errorcluster, "FPGA VI Reference Out"=w1519:T19)
        n1036 = xnode "Read/Write Control"("FPGA VI Reference In"=w1519, "error in"=w1518, "FB On/Off Set 1"=w1514, "FB On/Off Set 2"=w1511) -> ("error out"=w1517:errorcluster)  [unwired: 1 out]
      }
      event "Load parameters": Value Change {
        n1037 = event-data() -> ()  [unwired: 7 out]
        n1038 = property on="Saved AOD Raster Scan Parameter Sets" class="Arr (strict)"() -> ("Index Values"=w1558:u32[])  [unwired: 2 in, 2 out]
        n1039 = Index Array(array=w1558, index=0) -> (element=w1555:u32)
        n1040 = local write "Load parameters"(FALSE ("Load parameters")) -> ()
        n1041 = Index Array(array="Saved AOD Raster Scan Parameter Sets", index=w1555) -> (element=w1554:T26)
        n1042 = Unbundle By Name(w1554) -> ("Scan Range AOD (nm) 2"=w1553:dbl, "Step Size AOD (nm) 2"=w1552:dbl, "Scan Speed AOD (nm/s) 2"=w1551:dbl, "Number of scans (AOD) 2"=w1550:u16)
        n1043 = flat-sequence {
          tunnel: w1553 -> [w1561]
          tunnel: w1552 -> [w1560]
          tunnel: w1551 -> [w1559]
          tunnel: w1550 -> [w1562]
          frame #0 {
            n1044 = local write "Scan Speed (nm/s)"(w1559) -> ()
            n1045 = local write "Scan Range (nm)"(w1561) -> ()
            n1046 = local write "Step Size (nm)"(w1560) -> ()
          }
          frame #1 {
            n1047 = property on="Number of F/B Scans (AOD)" class="DigNum (strict)"("Val(Sgnl)"=w1562) -> ()  [unwired: 2 in, 2 out]
          }
        }
      }
      event "Trap 1 (ON/OFF)", "Trap 2 (ON/OFF)": Value Change {
        n1048 = event-data() -> ()  [unwired: 7 out]
        n1049 = property on="Trap 2 ON" class="Bool (strict)"("Val(Sgnl)"="Trap 2 (ON/OFF)") -> ()  [unwired: 2 in, 2 out]
        n1050 = property on="Trap 1 ON" class="Bool (strict)"("Val(Sgnl)"="Trap 1 (ON/OFF)") -> ()  [unwired: 2 in, 2 out]
      }
      event "DIO count 1 (ticks)", "DIO count 2 (ticks)", "DIO count 3 (ticks)", "Interlace", "Number Interlace Sets", "Not-Interlacing Set": Value Change {
        n1051 = event-data() -> ()  [unwired: 7 out]
        n1052 = local read "DIO count 3 (ticks)"() -> (w1575:u32)
        n1053 = local read "DIO count 1 (ticks)"() -> (w1577:u32)
        n1054 = local read "DIO count 2 (ticks)"() -> (w1576:u32)
        n1055 = To Unsigned Byte Integer(number="Not-Interlacing Set") -> (unsigned 8bit integer=w1566:u8)
        n1056 = Add(x=w1566, y=u8 1) -> (x+y=w1570:u8)
        n1057 = xnode "Read/Write Control"("FPGA VI Reference In"=w1581, "error in"=w1579, "DIO count 1 (ticks)"=w1577, "DIO count 2 (ticks)"=w1576, "DIO count 3 (ticks)"=w1575, "Interlace ON/OFF"="Interlace", "Number Interlace Cycles"="Number Interlace Sets", "Interlace Off Parameters"=w1570) -> ("error out"=w1580:errorcluster)  [unwired: 1 out]
        n1058 = Build Array(w1577, w1576, w1575) -> (w1568:u32[])
        n1059 = Split 1D Array(array=w1568, index="Number Interlace Sets") -> (first subarray=w1578:u32[])  [unwired: 1 out]
        n1060 = Index Array(array=w1568, index=w1566) -> (element=w1567:u32)
        n1061 = Add Array Elements(numeric array=w1578) -> (sum=w1572:u32)
        n1062 = Select(t=w1572, s="Interlace", f=w1567) -> (s? t:f=→"Total Counts (ticks)":u32)
      }
      event "Reset Feedback": Value Change {
        n1063 = event-data() -> ()  [unwired: 7 out]
        n1064 = Unbundle By Name("Reset Feedback") -> ("Set 1"=w1585:bool, "Set 2"=w1584:bool)
        n1065 = xnode "Read/Write Control"("FPGA VI Reference In"=w1587, "error in"=w1582, "FB Reset Set 1"=w1585, "FB Reset Set 2"=w1584) -> ("error out"=w1583:errorcluster)  [unwired: 1 out]
      }
      event "PID Gains": Value Change {
        n1066 = event-data() -> ()  [unwired: 7 out]
        n1067 = Unbundle By Name("PID Gains") -> ("Set 1"=w1591:T14, "Set 2"=w1590:T14)
        n1068 = xnode "Read/Write Control"("FPGA VI Reference In"=w1592, "error in"=w1588, "FB Gains Set 1"=w1591, "FB Gains Set 2"=w1590) -> ("error out"=w1589:errorcluster)  [unwired: 1 out]
      }
      event "AI2 to Setpoint", "Setpoints (V)": Value Change {
        n1069 = event-data() -> ()  [unwired: 7 out]
        n1070 = xnode "Read/Write Control"("FPGA VI Reference In"=w1598, "error in"=w1594) -> ("FPGA VI Reference Out"=w1597:T19, "error out"=w1596:errorcluster, "AI2 Y Sum Set 1"=w1605:i16, "AI2 Y Sum Set 2"=w1604:i16)
        n1071 = Cluster To Array(cluster="AI2 to Setpoint") -> (array=w1608:bool[])
        n1072 = local read "AI2 (V)"() -> (w1606:cluster{"Set 1":dbl, "Set 2":dbl})
        n1073 = Or Array Elements(Boolean array=w1608) -> (logical OR=w1609:bool)
        n1074 = Bundle By Name(cluster=w1606, "Set 1"=w1605, "Set 2"=w1604) -> (w1603:cluster{"Set 1":dbl, "Set 2":dbl})
        n1075 = Divide(x=w1603, y=3276.7) -> (x/y=w1602:cluster{"Set 1":dbl, "Set 2":dbl})
        "AI2 (V)" <- w1602
        n1076 = case shown="True" w1609 {
          tunnel: [w1612 w1629] -> w1601
          tunnel: "AI2 to Setpoint" -> [_ w1625]
          tunnel: "Setpoints (V)" -> [w1613 w1628]
          tunnel: w1602 -> [_ w1622]
          frame False {
            n1077 = Multiply(x=3276.7, y=w1613) -> (x*y=w1614:cluster{"Set 1":dbl, "Set 2":dbl})
            n1078 = To Word Integer(number=w1614) -> (16bit integer=w1612:cluster{"Set 1":i16, "Set 2":i16})
          }
          frame True {
            n1079 = Unbundle By Name(w1622) -> ("Set 1"=w1621:dbl, "Set 2"=w1620:dbl)
            n1080 = Unbundle By Name(w1628) -> ("Set 1"=w1627:dbl, "Set 2"=w1626:dbl)
            n1081 = Unbundle By Name(w1625) -> ("Set 1"=w1624:bool, "Set 2"=w1623:bool)
            n1082 = Select(t=w1621, s=w1624, f=w1627) -> (s? t:f=w1619:dbl)
            n1083 = Select(t=w1620, s=w1623, f=w1626) -> (s? t:f=w1618:dbl)
            n1084 = Bundle By Name(cluster=w1628, "Set 1"=w1619, "Set 2"=w1618) -> (w1616:cluster{"Set 1":dbl, "Set 2":dbl})
            n1085 = local write "Setpoints (V)"(w1616) -> ()
            n1086 = Multiply(x=3276.7, y=w1616) -> (x*y=w1617:cluster{"Set 1":dbl, "Set 2":dbl})
            n1087 = To Word Integer(number=w1617) -> (16bit integer=w1629:cluster{"Set 1":i16, "Set 2":i16})
          }
        }
        n1088 = Unbundle By Name(w1601) -> ("Set 1"=w1600:i16, "Set 2"=w1599:i16)
        n1089 = xnode "Read/Write Control"("FPGA VI Reference In"=w1597, "error in"=w1596, "FB Setpoint Set 1"=w1600, "FB Setpoint Set 2"=w1599) -> ("error out"=w1595:errorcluster)  [unwired: 1 out]
      }
      event "Invert GI": Value Change {
        n1090 = event-data() -> ()  [unwired: 7 out]
        n1091 = xnode "Read/Write Control"("FPGA VI Reference In"=w1634, "error in"=w1632, "Invert GI"="Invert GI", "Invert GI 2"="Invert GI") -> ("error out"=w1633:errorcluster)  [unwired: 1 out]
      }
      event "Green FB Setpoint (mV)", "Green FB Gains", "Green FB On/Off", "Current When FB OFF (%)", "Green int current ON count adj": Value Change {
        n1092 = event-data() -> ()  [unwired: 7 out]
        n1093 = local read "Green FB Setpoint (mV)"() -> (w1641:dbl)
        n1094 = local read "Current When FB OFF (%)"() -> (w1644:dbl)
        n1095 = Multiply(x=w1641, y=3.2767) -> (x*y=w1640:dbl)
        n1096 = Multiply(x=w1644, y=655.35) -> (x*y=w1645:dbl)
        n1097 = To Unsigned Word Integer(number=w1645) -> (unsigned 16bit integer=w1643:u16)
        n1098 = local read "Green int current ON count adj"() -> (w1648:u32)
        n1099 = local read "Green FB Gains"() -> (w1647:T14)
        n1100 = local read "Green Laser ON/Interlacing"() -> (w1638:bool)
        n1101 = local read "Green laser mode"() -> (w1637:enum32{"Laser ON", "Laser OFF", "Interlace"})
        n1102 = local read "Green FB On/Off"() -> (w1649:bool)
        n1103 = Equal?(x=w1637, y=enum32{"Laser ON", "Laser OFF", "Interlace"}."Interlace") -> (x = y?=w1635:bool)
        n1104 = Compound Arithmetic op=AND(w1635, w1649, w1638) -> (w1639:bool)
        n1105 = xnode "Read/Write Control"("FPGA VI Reference In"=w1652, "error in"=w1651, "Green FB Setpoint"=w1640, "Green FB On/Off"=w1639, "Current Out"=w1643, "Green int current ON count adj"=w1648, "Green FB Gains"=w1647) -> ("error out"=w1650:errorcluster)  [unwired: 1 out]
      }
      event "Green laser mode", "Green Laser ON/Interlacing": Value Change {
        n1106 = event-data() -> ()  [unwired: 7 out]
        n1107 = case shown="True" "Green Laser ON/Interlacing" {
          tunnel: "Green laser mode" -> [_ w1666]
          tunnel: [enum32{"Laser ON", "Laser OFF", "Interlace"}."Laser OFF" ("Green laser mode") w1666] -> w1654
          tunnel: [FALSE w1662] -> w1653
          frame False {
          }
          frame True {
            n1108 = local read "Green FB On/Off"() -> (w1663:bool)
            n1109 = Equal?(x=w1666, y=enum32{"Laser ON", "Laser OFF", "Interlace"}."Interlace") -> (x = y?=w1664:bool)
            n1110 = And(x=w1664, y=w1663) -> (x .and. y?=w1662:bool)
          }
        }
        n1111 = xnode "Read/Write Control"("FPGA VI Reference In"=w1659, "error in"=w1657, "Operating Mode"=w1654, "Operating Mode 2"=w1654, "Green FB On/Off"=w1653) -> ("error out"=w1658:errorcluster)  [unwired: 1 out]
      }
      event "Test ttrig": Value Change {
        n1112 = event-data() -> ()  [unwired: 7 out]
        n1113 = xnode "Read/Write Control"("FPGA VI Reference In"=w1670, "error in"=w1669, "TTrig?"=TRUE) -> ("error out"=w1668:errorcluster)  [unwired: 1 out]
      }
      event "Neg. TTrig FPGA": Value Change {
        n1114 = event-data() -> ()  [unwired: 7 out]
        n1115 = xnode "Read/Write Control"("FPGA VI Reference In"=w1674, "error in"=w1673, "TTrig Negate Pos"="Neg. TTrig FPGA") -> ()  [unwired: 2 out]
      }
      event "- phase (APD 1 Gate)", "+ phase (APD 1 Gate)": Value Change {
        n1116 = event-data() -> ()  [unwired: 7 out]
        n1117 = local read "Phase Adj. (APD 1 Gate)"() -> (w1675:i16)
        n1118 = Negate(x=w1675) -> (-x=w1683:i16)
        n1119 = Select(t=w1683, s="- phase (APD 1 Gate)", f=w1675) -> (s? t:f=w1682:i16)
        n1120 = Or(x="- phase (APD 1 Gate)", y="+ phase (APD 1 Gate)") -> (x .or. y?=w1678:bool)
        n1121 = xnode "Read/Write Control"("FPGA VI Reference In"=w1685, "error in"=w1684, "Phase count adjustment (APD 1 Gate)"=w1682) -> ("FPGA VI Reference Out"=w1680:T19, "error out"=w1681:errorcluster)
        n1122 = xnode "Read/Write Control"("FPGA VI Reference In"=w1680, "error in"=w1681, "+ phase (APD 1 Gate)"=w1678) -> ("error out"=w1679:errorcluster)  [unwired: 1 out]
      }
      event "+ phase (APD 2 Gate)", "- phase (APD 2 Gate)": Value Change {
        n1123 = event-data() -> ()  [unwired: 7 out]
        n1124 = local read "Phase Adj. (APD 2 Gate)"() -> (w1686:i16)
        n1125 = Negate(x=w1686) -> (-x=w1694:i16)
        n1126 = Select(t=w1694, s="- phase (APD 2 Gate)", f=w1686) -> (s? t:f=w1693:i16)
        n1127 = Or(x="- phase (APD 2 Gate)", y="+ phase (APD 2 Gate)") -> (x .or. y?=w1689:bool)
        n1128 = xnode "Read/Write Control"("FPGA VI Reference In"=w1696, "error in"=w1695, "Phase count adjustment (APD 2 Gate)"=w1693) -> ("FPGA VI Reference Out"=w1691:T19, "error out"=w1692:errorcluster)
        n1129 = xnode "Read/Write Control"("FPGA VI Reference In"=w1691, "error in"=w1692, "+ phase (APD 2 Gate)"=w1689) -> ("error out"=w1690:errorcluster)  [unwired: 1 out]
      }
      event "Phase Adj. (APD Acq)", "+ phase (APD Acq)", "- phase (APD Acq)": Value Change {
        n1130 = event-data() -> ()  [unwired: 7 out]
        n1131 = local read "Phase Adj. (APD Acq)"() -> (w1699:i16)
        n1132 = Negate(x=w1699) -> (-x=w1705:i16)
        n1133 = Select(t=w1705, s="+ phase (APD Acq)", f=w1699) -> (s? t:f=w1704:i16)
        n1134 = Or(x="+ phase (APD Acq)", y="- phase (APD Acq)") -> (x .or. y?=w1700:bool)
        n1135 = xnode "Read/Write Control"("FPGA VI Reference In"=w1707, "error in"=w1706, "Phase Count Adjustment (APD Acq)"=w1704) -> ("FPGA VI Reference Out"=w1702:T19, "error out"=w1703:errorcluster)
        n1136 = xnode "Read/Write Control"("FPGA VI Reference In"=w1702, "error in"=w1703, "+ phase (APD Acq)"=w1700) -> ("error out"=w1701:errorcluster)  [unwired: 1 out]
      }
      event "Phase adj. (GI)", "+ phase (GI)", "- phase (GI)": Value Change {
        n1137 = event-data() -> ()  [unwired: 7 out]
        n1138 = Negate(x="Phase adj. (GI)") -> (-x=w1716:i16)
        n1139 = Select(t=w1716, s="+ phase (GI)", f="Phase adj. (GI)") -> (s? t:f=w1715:i16)
        n1140 = Or(x="+ phase (GI)", y="- phase (GI)") -> (x .or. y?=w1711:bool)
        n1141 = xnode "Read/Write Control"("FPGA VI Reference In"=w1718, "error in"=w1717, "Phase count adjustment (GI)"=w1715) -> ("FPGA VI Reference Out"=w1713:T19, "error out"=w1714:errorcluster)
        n1142 = xnode "Read/Write Control"("FPGA VI Reference In"=w1713, "error in"=w1714, "+ phase (GI)"=w1711) -> ("error out"=w1712:errorcluster)  [unwired: 1 out]
      }
      event "Phase adj. (GI) 2", "+ phase (GI) 2", "- phase (GI) 2": Value Change {
        n1143 = event-data() -> ()  [unwired: 7 out]
        n1144 = Negate(x="Phase adj. (GI) 2") -> (-x=w1727:i16)
        n1145 = Select(t=w1727, s="+ phase (GI) 2", f="Phase adj. (GI) 2") -> (s? t:f=w1726:i16)
        n1146 = Or(x="+ phase (GI) 2", y="- phase (GI) 2") -> (x .or. y?=w1722:bool)
        n1147 = xnode "Read/Write Control"("FPGA VI Reference In"=w1729, "error in"=w1728, "Phase count adjustment (GI) 2"=w1726) -> ("FPGA VI Reference Out"=w1724:T19, "error out"=w1725:errorcluster)
        n1148 = xnode "Read/Write Control"("FPGA VI Reference In"=w1724, "error in"=w1725, "+ phase (GI) 2"=w1722) -> ("error out"=w1723:errorcluster)  [unwired: 1 out]
      }
      event "Phase adj. (Green FB)", "- phase (Green FB)", "+ phase (Green FB)": Value Change {
        n1149 = event-data() -> ()  [unwired: 7 out]
        n1150 = Negate(x="Phase adj. (Green FB)") -> (-x=w1738:i16)
        n1151 = Select(t=w1738, s="+ phase (Green FB)", f="Phase adj. (Green FB)") -> (s? t:f=w1737:i16)
        n1152 = Or(x="+ phase (Green FB)", y="- phase (Green FB)") -> (x .or. y?=w1733:bool)
        n1153 = xnode "Read/Write Control"("FPGA VI Reference In"=w1740, "error in"=w1739, "Phase count adjustment (Green FB)"=w1737) -> ("FPGA VI Reference Out"=w1735:T19, "error out"=w1736:errorcluster)
        n1154 = xnode "Read/Write Control"("FPGA VI Reference In"=w1735, "error in"=w1736, "+ phase (Green FB)"=w1733) -> ("error out"=w1734:errorcluster)  [unwired: 1 out]
      }
      event "Invert APD Gate", "APD Gate ON Count", "APD Gate OFF Count", "APD Gate", "APD Integration Time (s)", "APD 1 AO Mult.", "APD 2 AO Mult.", "On one out of X cycles": Value Change {
        n1155 = event-data() -> ()  [unwired: 7 out]
        n1156 = Add(x="GI Frequency, ON count", y="GI Frequency, OFF count") -> (x+y=w1744:u32)
        n1157 = Add(x="APD Gate ON Count", y="APD Gate OFF Count") -> (x+y=w1757:u32)
        n1158 = Multiply(x="On one out of X cycles", y=w1744) -> (x*y=w1741:u32)
        "Green FB Count" <- w1741
        n1159 = Subtract(x=w1741, y="GI Frequency, ON count") -> (x-y=w1742:u32)
        n1160 = Multiply(x=w1757, y="On one out of X cycles") -> (x*y=w1756:u32)
        n1161 = Subtract(x=w1756, y="APD Gate ON Count") -> (x-y=w1755:u32)
        n1162 = local read "DMA Update Period (s)"() -> (w1758:dbl)
        n1163 = Multiply(x="APD Integration Time (s)", y=40000000.0) -> (x*y=w1763:dbl)
        n1164 = Reciprocal(x="APD Integration Time (s)") -> (1/x=→"APD Acq Rate (Hz)":dbl)
        n1165 = To Unsigned Long Integer(number=w1763) -> (unsigned 32bit integer=w1747:u32)
        "APD Int. Count" <- w1747
        n1166 = xnode "Read/Write Control"("FPGA VI Reference In"=w1767, "error in"=w1766, "Invert APD Gate"="Invert APD Gate", "APD Gate ON Count"="APD Gate ON Count", "APD Gate OFF Count"=w1755, "APD Acq Rate Count"=w1747, "APD Gate Operating Mode"="APD Gate", "APD 1 AO scale factor"="APD 1 AO Mult.", "APD 2 AO scale factor"="APD 2 AO Mult.", "Green interlace ON count"="GI Frequency, ON count", "Green interlace OFF count"=w1742, "Green interlace ON count 2"="GI Frequency, ON count", "Green interlace OFF count 2"=w1742, "Green FB Count"=w1741) -> ("error out"=w1765:errorcluster)  [unwired: 1 out]
        n1167 = Divide(x=w1758, y="APD Integration Time (s)") -> (x/y=w1761:dbl)
        n1168 = Multiply(x=2.0, y=w1761) -> (x*y=w1760:dbl)
        n1169 = local write "APD Samples/FIFO Acq."(w1761) -> ()
        n1170 = local write "APD Elements/DMA read"(w1760) -> ()
      }
      event "Number of F/B Scans (AOD)", "Scan Speed (nm/s)", "Scan BD", "Initial delta (MHz)", "Step Size (nm)", "Scan Range (nm)": Value Change {
        w1829 = 123.0  # AOM cal (nm/MHz)
        n1171 = event-data() -> ()  [unwired: 7 out]
        n1172 = local read "BD 1 Frequency 1 (MHz)"() -> (w1812:dbl)
        n1173 = local read "AOM X Cal (nm/MHz)"() -> (w1804:dbl)
        n1174 = local read "X RF Frequency Limits (MHz)"() -> (w1816:T16)
        n1175 = local read "Y RF Frequency Limits (MHz)"() -> (w1813:T16)
        n1176 = local read "BD 2 Frequency 1 (MHz)"() -> (w1818:dbl)
        n1177 = Negate(x="Scan Range (nm)") -> (-x=w1782:dbl)
        n1178 = Divide(x=w1782, y=w1804) -> (x/y=w1786:dbl)
        n1179 = Select(t=w1816, s="Scan BD", f=w1813) -> (s? t:f=w1815:T16)
        n1180 = Select(t=w1812, s="Scan BD", f=w1818) -> (s? t:f=w1817:dbl)
        n1181 = Unbundle By Name(w1815) -> ("Maximum"=w1824:dbl, "Minimum"=w1823:dbl)
        n1182 = Add(x=w1786, y=w1817) -> (x+y=w1821:dbl)
        n1183 = Divide(x=w1782, y="Step Size (nm)") -> (x/y=w1801:dbl)
        n1184 = Divide(x="Step Size (nm)", y=w1804) -> (x/y=w1810:dbl)
        n1185 = Absolute Value(x=w1801) -> (abs(x)=w1785:dbl)
        n1186 = Sign(1:w1782) -> (0:w1783:dbl)
        n1187 = In Range and Coerce(upper limit=w1824, x=w1821, lower limit=w1823) -> (coerced(x)=w1820:dbl, In Range?=w1822:bool)
        n1188 = To Unsigned Quad Integer(1:w1785) -> (0:w1800:u64)
        "Scan steps (AOD)" <- w1800
        n1189 = call "IR AOM freq to word.vi"("Frequency In (MHz)"=w1810) -> ("Frequency Word Out (double)"=w1807:dbl)
        n1190 = Multiply(x=w1783, y=w1807) -> (x*y=w1784:dbl)
        n1191 = Subtract(x=w1821, y=w1820) -> (x-y=w1819:dbl)
        n1192 = To Quad Integer(1:w1784) -> (0:w1806:i64)
        "Incr. int (AOD)" <- w1806
        n1193 = Subtract(x=w1786, y=w1819) -> (x-y=w1805:dbl)
        "Scan Range (MHz)" <- w1805
        n1194 = Select(t=w1786, s=w1822, f=w1805) -> (s? t:f=w1825:dbl)
        n1195 = Multiply(x=w1805, y=w1804) -> (x*y=w1803:dbl)
        n1196 = Decrement(x=w1800) -> (x-1=w1853:u64)
        n1197 = Negate(x=w1803) -> (-x=w1799:dbl)
        n1198 = local write "Scan Range (nm)"(w1799) -> ()
        n1199 = Divide(x=w1825, y=w1853) -> (x/y=w1809:dbl)
        "Scan Increment (MHz)" <- w1809
        n1200 = call "IR AOM freq to word.vi"("Frequency In (MHz)"=w1809) -> ("Frequency Word Out (double)"=w1808:dbl)
        n1201 = Divide(x="Step Size (nm)", y="Scan Speed (nm/s)") -> (x/y=w1796:dbl)
        n1202 = To Quad Integer(1:w1808) -> ()  [unwired: 1 out]
        n1203 = local read "Number Interlace Sets"() -> (w1780:u8)
        n1204 = local read "AI Count (ticks)"() -> (w1781:u32)
        n1205 = local read "Total Counts (ticks)"() -> (w1779:u32)
        n1206 = local read "# Samples/trap"() -> (w1811:u32)
        n1207 = Multiply(x=w1781, y=w1780) -> (x*y=w1778:u32)
        n1208 = Divide(x=w1779, y=w1778) -> (x/y=w1777:dbl)
        n1209 = Select(t=w1812, s="Scan BD", f=w1818) -> (s? t:f=w1850:dbl)
        "Initial freq. (MHz)" <- w1850
        n1210 = Add(x=w1825, y=w1850) -> (x+y=→"Final freq. (MHz)":dbl)
        n1211 = Divide(x=w1779, y=40000000.0) -> (x/y=w1795:dbl)
        n1212 = Divide(x=w1796, y=w1795) -> (x/y=w1794:dbl)
        n1213 = To Unsigned Quad Integer(1:w1794) -> (0:w1769:u64)
        n1214 = Quotient & Remainder(x=w1769, y=u64 2) -> (x-y*floor(x/y)=w1773:u64)  [unwired: 1 out]
        n1215 = Equal?(x=w1773, y=u64 0) -> (x = y?=w1771:bool)
        n1216 = Decrement(x=w1769) -> (x-1=w1770:u64)
        n1217 = Select(t=w1769, s=w1771, f=w1770) -> (s? t:f=w1768:u64)
        "Cycles/step (AOD)" <- w1768
        n1218 = xnode "Read/Write Control"("FPGA VI Reference In"=w1861, "error in"=w1860, "Scan steps"=w1800, "Number of scans"="Number of F/B Scans (AOD)", "Cycles per step"=w1768, "Scan freq.  increment"=w1806, "Scan BD"="Scan BD") -> ("error out"=w1859:errorcluster)  [unwired: 1 out]
        n1219 = Multiply(x=w1800, y=w1768) -> (x*y=w1854:u64)
        n1220 = Multiply(x=w1854, y=u64 2) -> (x*y=w1776:u64)
        n1221 = Multiply(x=w1777, y=w1776) -> (x*y=w1775:dbl)
        "Data points/scan (f/b)" <- w1775
        n1222 = Multiply(x=w1775, y="Number of F/B Scans (AOD)") -> (x*y=w1857:dbl)
        "Data points/scans" <- w1857
        n1223 = Divide(x=w1857, y=w1811) -> (x/y=→"N sets should be saved":dbl)
        n1224 = Multiply(x=w1854, y=w1795) -> (x*y=w1793:dbl)
        "Time/Scan (s) (AOD)" <- w1793
        n1225 = Select(t=w1825, s="Scan BD", f=0.0) -> (s? t:f=w1851:dbl)
        n1226 = Select(t=0.0, s="Scan BD", f=w1825) -> (s? t:f=w1847:dbl)
        n1227 = local read "BD 2 Frequency 2 (MHz)"() -> (w1843:dbl)
        n1228 = local read "BD 1 Frequency 2 (MHz)"() -> (w1846:dbl)
        n1229 = Add(x=w1847, y=w1818) -> (x+y=w1844:dbl)
        n1230 = Add(x=w1812, y=w1851) -> (x+y=w1845:dbl)
        n1231 = Multiply(x=w1793, y=2.0) -> (x*y=w1792:dbl)
        n1232 = Multiply(x=w1792, y="Number of F/B Scans (AOD)") -> (x*y=w1789:dbl)
        n1233 = Divide(x=w1789, y=60.0) -> (x/y=→"Time to Finish All (min)":dbl)
        n1234 = Add(x="Trap 2 Bead Size (nm)", y="Trap 1 Bead Size (nm)") -> (x+y=w1833:dbl)
        n1235 = Divide(x=w1833, y=2.0) -> (x/y=w1827:dbl)
        n1236 = local read "Initial delta (MHz)"() -> (w1830:dbl)
        n1237 = Subtract(x=w1844, y=w1843) -> (x-y=w1841:dbl)
        n1238 = Subtract(x=w1845, y=w1846) -> (x-y=w1842:dbl)
        n1239 = Square(x=w1841) -> (x^2=w1840:dbl)
        n1240 = Square(x=w1842) -> (x^2=w1839:dbl)
        n1241 = Add(x=w1839, y=w1840) -> (x+y=w1838:dbl)
        n1242 = Square Root(x=w1838) -> (sqrt(x)=w1837:dbl)
        "Final delta (MHz)" <- w1837
        n1243 = Multiply(x=w1829, y=w1837) -> (x*y=w1836:dbl)
        n1244 = Multiply(x=w1830, y=w1829) -> (x*y=w1828:dbl)
        n1245 = Subtract(x=w1828, y=w1827) -> (x-y=→"Initial sep (nm)":dbl)
        n1246 = Subtract(x=w1836, y=w1827) -> (x-y=→"Final sep (nm)":dbl)
      }
      event "Freq or Amp switch first", "Swap F1 and F2", "Freq switch delay", "Amp switch delay": Value Change {
        n1247 = event-data() -> ()  [unwired: 7 out]
        n1248 = local read "Freq or Amp switch first"() -> (w1862:bool)
        n1249 = local read "Amp switch delay"() -> (w1863:u16)
        n1250 = local read "Freq switch delay"() -> (w1865:u16)
        n1251 = local read "Swap F1 and F2"() -> (w1864:bool)
        n1252 = xnode "Read/Write Control"("FPGA VI Reference In"=w1868, "error in"=w1867, "Freq switch delay"=w1865, "Swap F1 and F2"=w1864, "Amp switch delay"=w1863, "Freq or Amp switch first"=w1862) -> ("error out"=w1866:errorcluster)  [unwired: 1 out]
      }
      event "Scan steps (MCL)", "Number of scans (MCL)", "Scan Range (V)\n(of steps)", "2D or 1D Scan", "N APD Samp/step", "Fast Scan Dir", "Continuous MCL Scanning", "Scan lines (y)": Value Change {
        w1870 = 32767.0 ("y")
        n1253 = event-data() -> ()  [unwired: 7 out]
        n1254 = Select(t="Scan lines (y)", s="2D or 1D Scan", f="Number of scans (MCL)") -> (s? t:f=w1875:u64)
